vi "RisData.vi"(0 "Action":T1(ring), 1 "Array No.":i32, 2 "Array Size / Index":i32, 3 "Data IN":dbl format="%.2f", 4 "Array IN":dbl[](array[numeric]) format="%.2f") -> (5 "Data OUT":dbl format="%.2f", 6 "Array OUT":dbl[](array[numeric]) format="%.2f")   [LabVIEW 2013]
doc: "Reset data arrays, or read/write array elements, or read entire\narrays.\nAction: 0 Reset arrays\n 1 Read array\n 2 Read array element\n 3 Write array element"
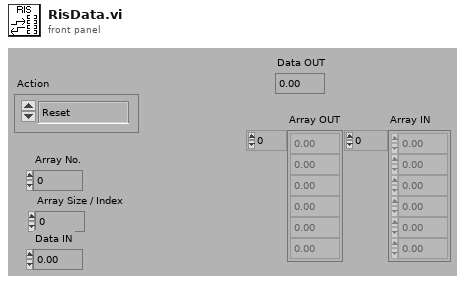
[diagram p1: front panel]
types:
  T1 = enum16{"Reset", "Read Array", "Read Element", "Write Element", "Write Array", "Add Element", "Add Array"}
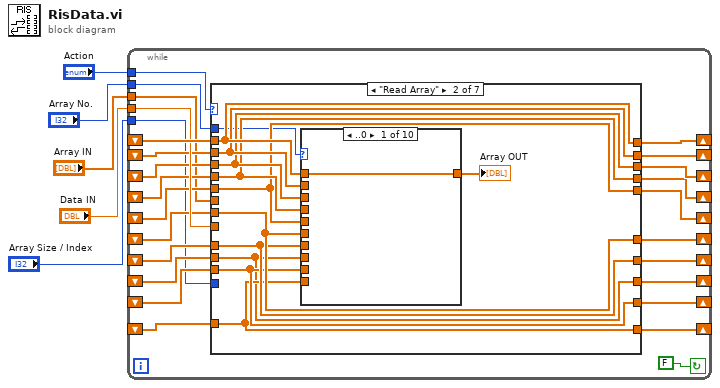
[diagram p0: block diagram]
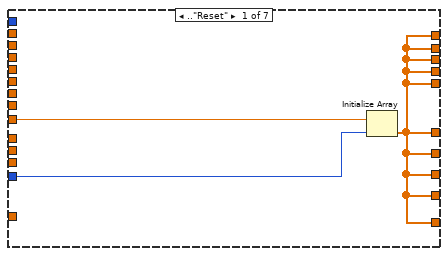
[diagram p2: hidden frame]
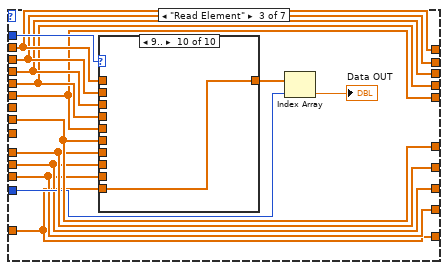
[diagram p12: hidden frame]
diagram:
  n1 = while {
    shift-left: _ -> [w11]
    shift-right: [w10] -> _
    tunnel: "Array No." -> [w12]
    shift-left: _ -> [w13]
    shift-right: [w21] -> _
    shift-left: _ -> [w14]
    shift-right: [w9] -> _
    shift-left: _ -> [w15]
    shift-right: [w22] -> _
    shift-left: _ -> [w16]
    shift-right: [w23] -> _
    shift-left: _ -> [w17]
    shift-right: [w24] -> _
    shift-left: _ -> [w18]
    shift-right: [w25] -> _
    shift-left: _ -> [w19]
    shift-right: [w26] -> _
    shift-left: _ -> [w20]
    shift-right: [w27] -> _
    tunnel: "Data IN" -> [w29]
    tunnel: "Array Size / Index" -> [w7]
    tunnel: "Action" -> [w31]
    shift-left: _ -> [w30]
    shift-right: [w28] -> _
    tunnel: "Array IN" -> [w6]
    stop <- FALSE continue-if-true
    n2 = case shown="\"Read Array\"" w31 {
      tunnel: [w34 w46 w69 w99 w245 w405 w538] -> w28
      tunnel: w30 -> [_ w46 w69 w103 w256 w407 w539]
      tunnel: w7 -> [w32 _ w61 w100 w254 _ _]
      tunnel: w29 -> [w33 _ _ w101 _ w406 _]
      tunnel: [w34 w44 w67 w90 w244 w403 w537] -> w27
      tunnel: [w34 w43 w66 w89 w243 w400 w536] -> w26
      tunnel: [w34 w42 w65 w88 w242 w399 w535] -> w25
      tunnel: [w34 w41 w64 w85 w241 w397 w534] -> w24
      tunnel: [w34 w40 w63 w83 w240 w396 w533] -> w23
      tunnel: [w34 w39 w62 w87 w239 w395 w532] -> w22
      tunnel: [w34 w35 w59 w81 w238 w394 w531] -> w9
      tunnel: [w34 w38 w58 w82 w237 w388 w530] -> w21
      tunnel: w20 -> [_ w44 w67 w98 w255 w404 w540]
      tunnel: w19 -> [_ w43 w66 w97 w253 w402 w541]
      tunnel: w18 -> [_ w42 w65 w96 w252 w401 w542]
      tunnel: w17 -> [_ w41 w64 w95 w251 w398 w543]
      tunnel: w16 -> [_ w40 w63 w84 w250 w393 w545]
      tunnel: w15 -> [_ w39 w62 w94 w249 w392 w546]
      tunnel: w14 -> [_ w35 w59 w93 w248 w391 w547]
      tunnel: w13 -> [_ w38 w58 w92 w247 w390 w548]
      tunnel: w12 -> [_ w37 w70 w102 w235 w408 w550]
      tunnel: w11 -> [_ w36 w57 w91 w246 w389 w549]
      tunnel: [w34 w36 w57 w86 w236 w387 w529] -> w10
      tunnel: w6 -> [_ _ _ _ w234 _ w544]
      frame .."Reset" {
        n3 = Initialize Array(w33, w32) -> (w34:dbl[])
      }
      frame "Read Array" {
        n4 = case shown="..0" w37 {
          tunnel: w46 -> [w47 _ _ _ _ _ _ _ _ _]
          tunnel: [w47 w48 w49 w50 w51 w52 w53 w54 w55 w56] -> w45
          tunnel: w44 -> [_ w48 _ _ _ _ _ _ _ _]
          tunnel: w43 -> [_ _ w49 _ _ _ _ _ _ _]
          tunnel: w42 -> [_ _ _ w50 _ _ _ _ _ _]
          tunnel: w41 -> [_ _ _ _ w51 _ _ _ _ _]
          tunnel: w40 -> [_ _ _ _ _ w52 _ _ _ _]
          tunnel: w39 -> [_ _ _ _ _ _ w53 _ _ _]
          tunnel: w35 -> [_ _ _ _ _ _ _ w54 _ _]
          tunnel: w38 -> [_ _ _ _ _ _ _ _ w55 _]
          tunnel: w36 -> [_ _ _ _ _ _ _ _ _ w56]
          frame ..0 {
          }
          frame 1 {
          }
          frame 2 {
          }
          frame 3 {
          }
          frame 4 {
          }
          frame 5 {
          }
          frame 6 {
          }
          frame 7 {
          }
          frame 8 {
          }
          frame 9.. {
          }
        }
        "Array OUT" <- w45
      }
      frame "Read Element" {
        n5 = case shown="9.." w70 {
          tunnel: w69 -> [w71 _ _ _ _ _ _ _ _ _]
          tunnel: [w71 w72 w73 w74 w75 w76 w77 w78 w79 w80] -> w68
          tunnel: w67 -> [_ w72 _ _ _ _ _ _ _ _]
          tunnel: w66 -> [_ _ w73 _ _ _ _ _ _ _]
          tunnel: w65 -> [_ _ _ w74 _ _ _ _ _ _]
          tunnel: w64 -> [_ _ _ _ w75 _ _ _ _ _]
          tunnel: w63 -> [_ _ _ _ _ w76 _ _ _ _]
          tunnel: w62 -> [_ _ _ _ _ _ w77 _ _ _]
          tunnel: w59 -> [_ _ _ _ _ _ _ w78 _ _]
          tunnel: w58 -> [_ _ _ _ _ _ _ _ w79 _]
          tunnel: w57 -> [_ _ _ _ _ _ _ _ _ w80]
          frame ..0 {
          }
          frame 1 {
          }
          frame 2 {
          }
          frame 3 {
          }
          frame 4 {
          }
          frame 5 {
          }
          frame 6 {
          }
          frame 7 {
          }
          frame 8 {
          }
          frame 9.. {
          }
        }
        n6 = Index Array(array=w68, index=w61) -> (element=→"Data OUT":dbl)
      }
      frame "Write Element" {
        n7 = case shown="9.." w102 {
          tunnel: w103 -> [w114 w129 w142 w155 w168 w181 w194 w207 w220 w233]
          tunnel: w101 -> [w116 w128 w138 w150 w162 w174 w186 w198 w211 w224]
          tunnel: w100 -> [w115 w127 w137 w149 w161 w173 w185 w197 w210 w221]
          tunnel: [w113 w129 w142 w155 w168 w181 w194 w207 w220 w233] -> w99
          tunnel: w98 -> [w111 w126 w141 w154 w167 w180 w193 w206 w219 w232]
          tunnel: w97 -> [w110 w124 w140 w153 w166 w179 w192 w205 w218 w231]
          tunnel: w96 -> [w109 w123 w136 w152 w165 w178 w191 w204 w217 w230]
          tunnel: w95 -> [w108 w122 w135 w148 w164 w177 w190 w203 w216 w229]
          tunnel: w94 -> [w107 w120 w133 w146 w159 w172 w188 w201 w214 w227]
          tunnel: w93 -> [w106 w119 w132 w145 w158 w171 w184 w200 w213 w226]
          tunnel: w92 -> [w105 w118 w131 w144 w157 w170 w183 w196 w212 w225]
          tunnel: w91 -> [w104 w117 w130 w143 w156 w169 w182 w195 w208 w223]
          tunnel: [w106 w119 w132 w145 w158 w171 w184 w199 w213 w226] -> w81
          tunnel: [w104 w117 w130 w143 w156 w169 w182 w195 w208 w222] -> w86
          tunnel: [w112 w121 w134 w147 w160 w175 w189 w202 w215 w228] -> w83
          tunnel: w84 -> [w112 w121 w134 w147 w160 w176 w189 w202 w215 w228]
          tunnel: [w109 w123 w136 w151 w165 w178 w191 w204 w217 w230] -> w88
          tunnel: [w105 w118 w131 w144 w157 w170 w183 w196 w209 w225] -> w82
          tunnel: [w111 w125 w141 w154 w167 w180 w193 w206 w219 w232] -> w90
          tunnel: [w110 w124 w139 w153 w166 w179 w192 w205 w218 w231] -> w89
          tunnel: [w108 w122 w135 w148 w163 w177 w190 w203 w216 w229] -> w85
          tunnel: [w107 w120 w133 w146 w159 w172 w187 w201 w214 w227] -> w87
          frame ..0 {
            n8 = Replace Array Subset(array=w114, new element=w116, index=w115) -> (w113:dbl[])
          }
          frame 1 {
            n9 = Replace Array Subset(array=w126, new element=w128, index=w127) -> (w125:dbl[])
          }
          frame 2 {
            n10 = Replace Array Subset(array=w140, new element=w138, index=w137) -> (w139:dbl[])
          }
          frame 3 {
            n11 = Replace Array Subset(array=w152, new element=w150, index=w149) -> (w151:dbl[])
          }
          frame 4 {
            n12 = Replace Array Subset(array=w164, new element=w162, index=w161) -> (w163:dbl[])
          }
          frame 5 {
            n13 = Replace Array Subset(array=w176, new element=w174, index=w173) -> (w175:dbl[])
          }
          frame 6 {
            n14 = Replace Array Subset(array=w188, new element=w186, index=w185) -> (w187:dbl[])
          }
          frame 7 {
            n15 = Replace Array Subset(array=w200, new element=w198, index=w197) -> (w199:dbl[])
          }
          frame 8 {
            n16 = Replace Array Subset(array=w212, new element=w211, index=w210) -> (w209:dbl[])
          }
          frame 9.. {
            n17 = Replace Array Subset(array=w223, new element=w224, index=w221) -> (w222:dbl[])
          }
        }
      }
      frame "Write Array" {
        n18 = case shown="..0" w235 {
          tunnel: w256 -> [w267 w282 w295 w308 w321 w334 w347 w360 w373 w386]
          tunnel: w234 -> [w269 w281 w291 w303 w315 w327 w339 w351 w364 w377]
          tunnel: w254 -> [w268 w280 w290 w302 w314 w326 w338 w350 w363 w374]
          tunnel: [w266 w282 w295 w308 w321 w334 w347 w360 w373 w386] -> w245
          tunnel: w255 -> [w264 w279 w294 w307 w320 w333 w346 w359 w372 w385]
          tunnel: w253 -> [w263 w277 w293 w306 w319 w332 w345 w358 w371 w384]
          tunnel: w252 -> [w262 w276 w289 w305 w318 w331 w344 w357 w370 w383]
          tunnel: w251 -> [w261 w275 w288 w301 w317 w330 w343 w356 w369 w382]
          tunnel: w249 -> [w260 w273 w286 w299 w312 w325 w341 w354 w367 w380]
          tunnel: w248 -> [w259 w272 w285 w298 w311 w324 w337 w353 w366 w379]
          tunnel: w247 -> [w258 w271 w284 w297 w310 w323 w336 w349 w365 w378]
          tunnel: w246 -> [w257 w270 w283 w296 w309 w322 w335 w348 w361 w376]
          tunnel: [w259 w272 w285 w298 w311 w324 w337 w352 w366 w379] -> w238
          tunnel: [w257 w270 w283 w296 w309 w322 w335 w348 w361 w375] -> w236
          tunnel: [w265 w274 w287 w300 w313 w328 w342 w355 w368 w381] -> w240
          tunnel: w250 -> [w265 w274 w287 w300 w313 w329 w342 w355 w368 w381]
          tunnel: [w262 w276 w289 w304 w318 w331 w344 w357 w370 w383] -> w242
          tunnel: [w258 w271 w284 w297 w310 w323 w336 w349 w362 w378] -> w237
          tunnel: [w264 w278 w294 w307 w320 w333 w346 w359 w372 w385] -> w244
          tunnel: [w263 w277 w292 w306 w319 w332 w345 w358 w371 w384] -> w243
          tunnel: [w261 w275 w288 w301 w316 w330 w343 w356 w369 w382] -> w241
          tunnel: [w260 w273 w286 w299 w312 w325 w340 w354 w367 w380] -> w239
          frame ..0 {
            n19 = Replace Array Subset(array=w267, new element=w269, index=w268) -> (w266:dbl[])
          }
          frame 1 {
            n20 = Replace Array Subset(array=w279, new element=w281, index=w280) -> (w278:dbl[])
          }
          frame 2 {
            n21 = Replace Array Subset(array=w293, new element=w291, index=w290) -> (w292:dbl[])
          }
          frame 3 {
            n22 = Replace Array Subset(array=w305, new element=w303, index=w302) -> (w304:dbl[])
          }
          frame 4 {
            n23 = Replace Array Subset(array=w317, new element=w315, index=w314) -> (w316:dbl[])
          }
          frame 5 {
            n24 = Replace Array Subset(array=w329, new element=w327, index=w326) -> (w328:dbl[])
          }
          frame 6 {
            n25 = Replace Array Subset(array=w341, new element=w339, index=w338) -> (w340:dbl[])
          }
          frame 7 {
            n26 = Replace Array Subset(array=w353, new element=w351, index=w350) -> (w352:dbl[])
          }
          frame 8 {
            n27 = Replace Array Subset(array=w365, new element=w364, index=w363) -> (w362:dbl[])
          }
          frame 9.. {
            n28 = Replace Array Subset(array=w376, new element=w377, index=w374) -> (w375:dbl[])
          }
        }
      }
      frame "Add Element" {
        n29 = case shown="1" w408 {
          tunnel: w407 -> [w420 w429 w441 w453 w465 w477 w489 w501 w513 w525]
          tunnel: w406 -> [w419 w431 w444 w454 w468 w478 w492 w504 w515 w527]
          tunnel: [w418 w429 w441 w453 w465 w477 w489 w501 w513 w525] -> w405
          tunnel: w404 -> [w417 w432 w440 w452 w464 w476 w488 w500 w512 w524]
          tunnel: [w417 w430 w440 w452 w464 w476 w488 w500 w512 w524] -> w403
          tunnel: w402 -> [w416 w428 w443 w451 w463 w475 w487 w499 w511 w523]
          tunnel: w401 -> [w415 w427 w433 w456 w462 w474 w486 w498 w510 w522]
          tunnel: [w416 w428 w442 w451 w463 w475 w487 w499 w511 w523] -> w400
          tunnel: [w415 w427 w433 w455 w462 w474 w486 w498 w510 w522] -> w399
          tunnel: w398 -> [w414 w426 w434 w450 w467 w473 w485 w497 w509 w521]
          tunnel: [w414 w426 w434 w450 w466 w473 w485 w497 w509 w521] -> w397
          tunnel: [w413 w425 w435 w449 w461 w479 w484 w496 w508 w520] -> w396
          tunnel: w393 -> [w413 w425 w435 w449 w461 w480 w484 w496 w508 w520]
          tunnel: w392 -> [w412 w424 w436 w448 w460 w472 w491 w495 w507 w519]
          tunnel: [w412 w424 w436 w448 w460 w472 w490 w495 w507 w519] -> w395
          tunnel: [w411 w423 w437 w447 w459 w471 w483 w503 w506 w518] -> w394
          tunnel: w391 -> [w411 w423 w437 w447 w459 w471 w483 w502 w506 w518]
          tunnel: w390 -> [w410 w422 w438 w446 w458 w470 w482 w494 w516 w517]
          tunnel: w389 -> [w409 w421 w439 w445 w457 w469 w481 w493 w505 w528]
          tunnel: [w410 w422 w438 w446 w458 w470 w482 w494 w514 w517] -> w388
          tunnel: [w409 w421 w439 w445 w457 w469 w481 w493 w505 w526] -> w387
          frame ..0 {
            n30 = Build Array (concatenate)(w420, w419) -> (w418:dbl[])
          }
          frame 1 {
            n31 = Build Array (concatenate)(w432, w431) -> (w430:dbl[])
          }
          frame 2 {
            n32 = Build Array (concatenate)(w443, w444) -> (w442:dbl[])
          }
          frame 3 {
            n33 = Build Array (concatenate)(w456, w454) -> (w455:dbl[])
          }
          frame 4 {
            n34 = Build Array (concatenate)(w467, w468) -> (w466:dbl[])
          }
          frame 5 {
            n35 = Build Array (concatenate)(w480, w478) -> (w479:dbl[])
          }
          frame 6 {
            n36 = Build Array (concatenate)(w491, w492) -> (w490:dbl[])
          }
          frame 7 {
            n37 = Build Array (concatenate)(w502, w504) -> (w503:dbl[])
          }
          frame 8 {
            n38 = Build Array (concatenate)(w516, w515) -> (w514:dbl[])
          }
          frame 9.. {
            n39 = Build Array (concatenate)(w528, w527) -> (w526:dbl[])
          }
        }
      }
      frame "Add Array".. {
        n40 = case shown="1" w550 {
          tunnel: w549 -> [w551 w574 w581 w598 w608 w621 w634 w646 w655 w670]
          tunnel: w548 -> [w552 w573 w580 w597 w607 w620 w633 w645 w658 w667]
          tunnel: w547 -> [w553 w572 w579 w596 w606 w619 w632 w644 w654 w666]
          tunnel: w546 -> [w554 w571 w578 w595 w605 w618 w631 w636 w653 w665]
          tunnel: w545 -> [w555 w570 w577 w594 w604 w611 w628 w635 w652 w664]
          tunnel: w544 -> [w562 w567 w586 w593 w610 w622 w630 w640 w657 w669]
          tunnel: w543 -> [w556 w569 w576 w587 w609 w616 w627 w637 w651 w663]
          tunnel: w542 -> [w557 w568 w575 w592 w602 w615 w623 w638 w650 w662]
          tunnel: w541 -> [w558 w563 w584 w588 w601 w614 w624 w641 w649 w661]
          tunnel: w540 -> [w560 w564 w582 w589 w600 w613 w625 w642 w648 w660]
          tunnel: w539 -> [w559 w565 w583 w590 w599 w612 w626 w643 w647 w659]
          tunnel: [w561 w565 w583 w590 w599 w612 w626 w643 w647 w659] -> w538
          tunnel: [w560 w566 w582 w589 w600 w613 w625 w642 w648 w660] -> w537
          tunnel: [w558 w563 w585 w588 w601 w614 w624 w641 w649 w661] -> w536
          tunnel: [w557 w568 w575 w591 w602 w615 w623 w638 w650 w662] -> w535
          tunnel: [w556 w569 w576 w587 w603 w616 w627 w637 w651 w663] -> w534
          tunnel: [w555 w570 w577 w594 w604 w617 w628 w635 w652 w664] -> w533
          tunnel: [w554 w571 w578 w595 w605 w618 w629 w636 w653 w665] -> w532
          tunnel: [w553 w572 w579 w596 w606 w619 w632 w639 w654 w666] -> w531
          tunnel: [w552 w573 w580 w597 w607 w620 w633 w645 w656 w667] -> w530
          tunnel: [w551 w574 w581 w598 w608 w621 w634 w646 w655 w668] -> w529
          frame ..0 {
            n41 = Build Array (concatenate)(w559, w562) -> (w561:dbl[])
          }
          frame 1 {
            n42 = Build Array (concatenate)(w564, w567) -> (w566:dbl[])
          }
          frame 2 {
            n43 = Build Array (concatenate)(w584, w586) -> (w585:dbl[])
          }
          frame 3 {
            n44 = Build Array (concatenate)(w592, w593) -> (w591:dbl[])
          }
          frame 4 {
            n45 = Build Array (concatenate)(w609, w610) -> (w603:dbl[])
          }
          frame 5 {
            n46 = Build Array (concatenate)(w611, w622) -> (w617:dbl[])
          }
          frame 6 {
            n47 = Build Array (concatenate)(w631, w630) -> (w629:dbl[])
          }
          frame 7 {
            n48 = Build Array (concatenate)(w644, w640) -> (w639:dbl[])
          }
          frame 8 {
            n49 = Build Array (concatenate)(w658, w657) -> (w656:dbl[])
          }
          frame 9.. {
            n50 = Build Array (concatenate)(w670, w669) -> (w668:dbl[])
          }
        }
      }
    }
  }
